vi "pulsed_counts_new.vi"(5 "path in":path) -> (4 "timetags":u32[](graph), 6 "triggers":u32[](array[numeric]), 8 "stop measure":bool, 14 "path out":path, 15 "Error_out":errorcluster)   [LabVIEW 2018]
uses:
  <vilib>/DAQmx/read.llb/DAQmx Read (Counter 1D U32 1Chan NSamp).vi
  <vilib>/DAQmx/miscellaneous.llb/DAQmx Fill In Error Info.vi
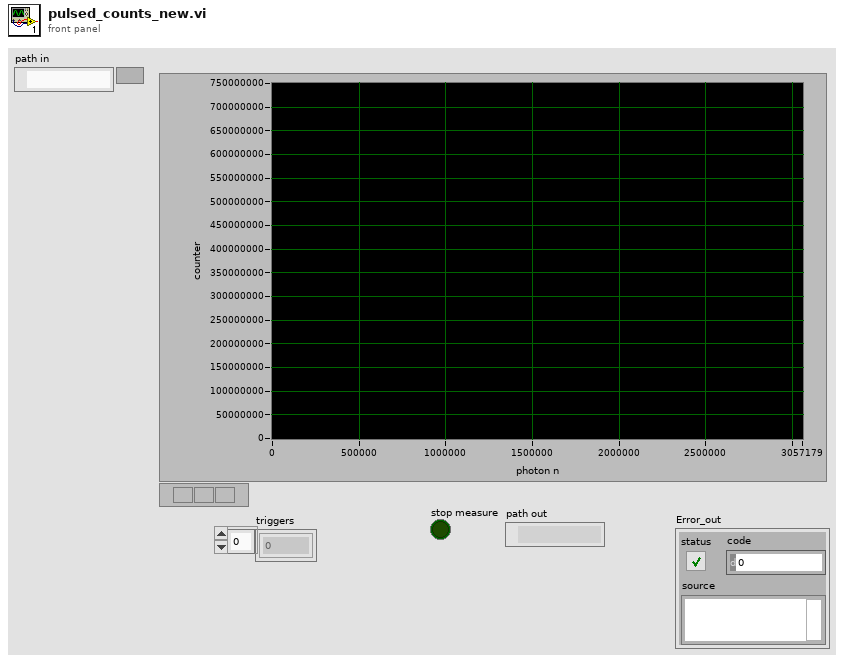
[diagram p1: front panel]
types:
  T1 = cluster{"Stopped":bool, "Reset":bool, "Running":bool, "Waiting":bool, "Scanning":bool}
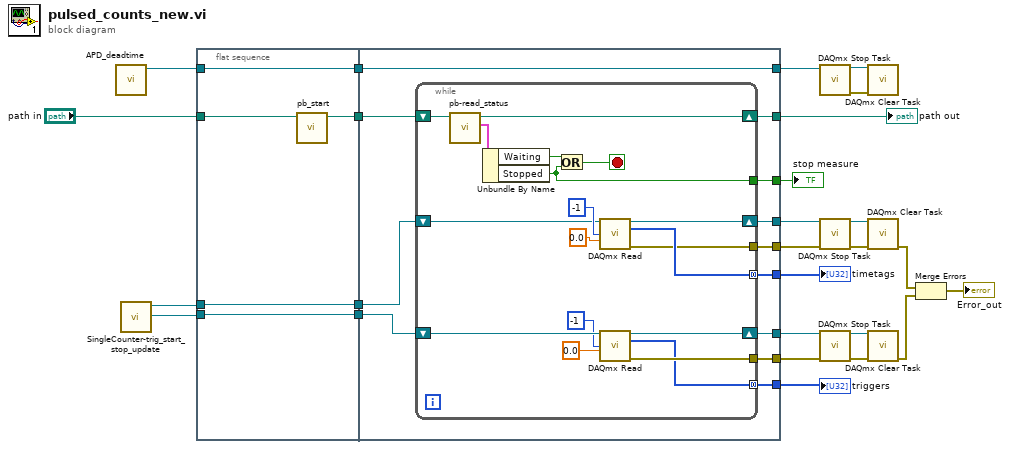
[diagram p0: block diagram]
diagram:
  n1 = call "APD_deadtime.vi"() -> ("filtered APD"=w21:refnum<k21>)  [unwired: 6 in, 1 out]
  n2 = call "SingleCounter-trig_start_stop_update.vi"() -> ("triggers_task"=w12:refnum<k21>, "APD_task"=w14:refnum<k21>)  [unwired: 8 in, 2 out]
  n3 = flat-sequence {
    tunnel: w21 -> [w30]
    tunnel: w14 -> [w31]
    tunnel: [w31] -> w19
    tunnel: [w30] -> w18
    tunnel: "path in" -> [w27]
    tunnel: [w28] -> w17
    tunnel: [w29] -> w13
    tunnel: w12 -> [w29]
    tunnel: [w43] -> w22
    tunnel: [w41] -> w20
    tunnel: [w33] -> w1
    tunnel: [w40] -> w16
    tunnel: [w39] -> w15
    tunnel: [w37] -> w9
    tunnel: [w36] -> w8
    tunnel: [w35] -> w4
    tunnel: w13 -> [w38]
    tunnel: w17 -> [w34]
    tunnel: w18 -> [w41]
    tunnel: w19 -> [w42]
    tunnel: [w32] -> w2
    frame #0 {
      n4 = call "pb_start.vi"("path in"=w27) -> ("path out"=w28:path)  [unwired: 9 in, 1 out]
    }
    frame #1 {
      n5 = while {
        tunnel: [w60] -> w43 mode=concatenating
        tunnel: [w56] -> w39
        tunnel: [w51] -> w36
        tunnel: [w50] -> w35 mode=concatenating
        shift-right: [w57] -> w40
        shift-left: w42 -> [w59]
        shift-right: [w52] -> w37
        shift-left: w38 -> [w55]
        tunnel: [w44] -> w32
        shift-right: [w47] -> w33
        shift-left: w34 -> [w49]
        stop <- w46 stop-if-true
        n6 = call "pb-read_status.vi"("path in"=w49) -> ("status"=w48:T1, "path out"=w47:path)  [unwired: 8 in, 1 out]
        n7 = Unbundle By Name(w48) -> ("Waiting"=w45:bool, "Stopped"=w44:bool)
        n8 = Or(x=w45, y=w44) -> (x .or. y?=w46:bool)
        n9 = call-poly <vilib>:"DAQmx Read.vi"("task/channels in"=w59, "number of samples per channel"=-1, "timeout"=0.0) -> ("task out"=w57:refnum<k21>, "data"=w60:u32[], "error out"=w56:errorcluster)  [unwired: 10 in]
        n10 = call-poly <vilib>:"DAQmx Read.vi"("task/channels in"=w55, "number of samples per channel"=-1, "timeout"=0.0) -> ("task out"=w52:refnum<k21>, "data"=w50:u32[], "error out"=w51:errorcluster)  [unwired: 10 in]
      }
    }
  }
  n11 = call <vilib>:"DAQmx Stop Task.vi"("task/channels in"=w20) -> ("task out"=w24:refnum<k21>, "error out"=w23:errorcluster)  [unwired: 13 in]
  n12 = call <vilib>:"DAQmx Stop Task.vi"("task/channels in"=w16, "error in"=w15) -> ("task out"=w26:refnum<k21>, "error out"=w25:errorcluster)  [unwired: 12 in]
  n13 = call <vilib>:"DAQmx Stop Task.vi"("task/channels in"=w9, "error in"=w8) -> ("task out"=w11:refnum<k21>, "error out"=w10:errorcluster)  [unwired: 12 in]
  n14 = call <vilib>:"DAQmx Clear Task.vi"("task in"=w24, "error in"=w23) -> ()  [unwired: 13 in, 1 out]
  n15 = call <vilib>:"DAQmx Clear Task.vi"("task in"=w26, "error in"=w25) -> ("error out"=w6:errorcluster)  [unwired: 13 in]
  n16 = call <vilib>:"DAQmx Clear Task.vi"("task in"=w11, "error in"=w10) -> ("error out"=w7:errorcluster)  [unwired: 13 in]
  n17 = Merge Errors(w6, w7) -> (→"Error_out":errorcluster)
  "timetags" <- w22
  "triggers" <- w4
  "stop measure" <- w2
  "path out" <- w1
